vi "temp.vi"() -> ()   [LabVIEW 2014]
panel:
  out "Waveform Chart 2":dbl(graph)
  out "Waveform Chart":dbl(graph)
  in  "stop":bool
  out "MotorCommand":dbl
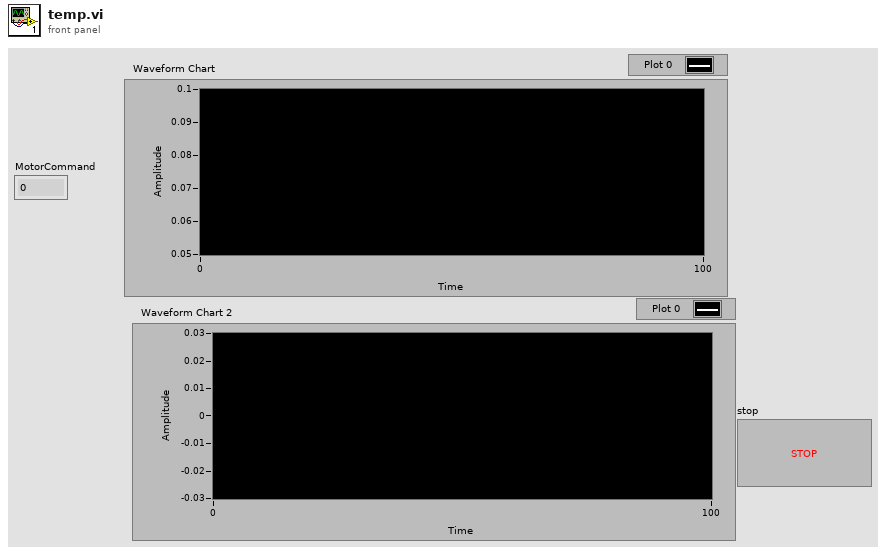
[diagram p1: front panel]
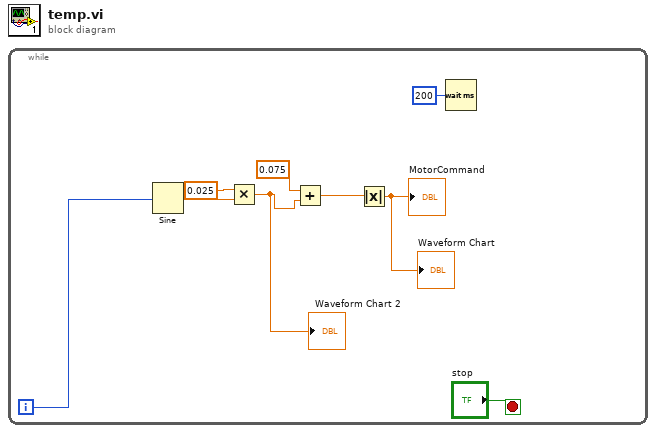
[diagram p0: block diagram]
diagram:
  n1 = while {
    i -> [w7]
    stop <- "stop" stop-if-true
    n2 = Sine(x=w7) -> (sin(x)=w4:dbl)
    n3 = Multiply(x=0.025, y=w4) -> (x*y=w1:dbl)
    "Waveform Chart 2" <- w1
    n4 = Add(x=0.075, y=w1) -> (x+y=w2:dbl)
    n5 = Absolute Value(x=w2) -> (abs(x)=→"MotorCommand" →"Waveform Chart":dbl)
    n6 = Wait (ms)(milliseconds to wait=u32 200) -> ()  [unwired: 1 out]
  }
